vi "database_connection_write_dev_MQTT_no_database.vi"(5 "ODBC data source name":string="amrc_monitoring", 6 "error in (no error)":errorcluster, 7 "G1?":u32, 8 "current time":timestamp, 9 "data 2":dbl[](array[numeric]), 10 "Machine Data":T4={"Zload"="", "Yload"="", "Xload"="", "path_position"="", "Fovr"="", "SspeedOvr"="", "Program Name"="", "Program status"="", "Block of code being executed"="", "Line of code"="", "Machine availability"="", "Emergency status"="", "Controller mode"="", "Tool_id"="UNAVAILABLE"}, 11 "Machine type":string) -> (3 "error out":errorcluster)   [LabVIEW 2017]
uses:
  <vilib>/regexp/Match Regular Expression.xnode
  mqtt Folder/src/class/mqtt/mqtt.lvclass
  mqtt Folder/src/class/mqtt/mqttTXqueue/mqttTXdataQueueFunction.ctl
  mqtt Folder/src/class/mqtt/mqttConfigFunction.ctl
  mqtt Folder/src/class/mqtt/mqttTXqueue/mqttRXsubscriptionEventFunction.ctl
  mqtt Folder/src/class/mqtt/mqttTypedef/mqttBroker.ctl
  mqtt Folder/src/class/mqtt/mqttTypedef/mqttConnectionFlags.ctl
  mqtt Folder/src/class/mqtt/mqttTypedef/mqttWillInformation.ctl
  <vilib>/addons/database/NI_Database_API.lvlib
  mqtt Folder/src/class/mqtt/mqttTypedef/mqttQOSlevel.ctl
  mqtt Folder/src/class/mqtt/mqttTypedef/mqttConnectionMeta.ctl
  mqtt Folder/src/class/mqtt/mqttTypedef/mqttConnectionStatus.ctl
panel:
  out "error out 3":errorcluster
  out "publishSuccess 2":bool=TRUE
  out "publishMessageID 2":u16 format="%02x"
  out "valueSent 2":string="14:19:17.238_"
  in  "connMeta 2":T1
  in  "topic 2":string="a/b"
  out "connStatus 2":T3
  out "sessionPresent 2":bool
  out "string":string="(timestamp,machine_status,g1,tool_id,force_acc_raw_data,spike_raw_data,spindle_load,spindle_speed,feed_rate,I,J,K,X,Y,Z,position_A,position_B ,Xload,Yload,Zload,Aload,Bload,program_number,accel_x_rms,accel_y_rms,accel_z_rms,force_x_rms,force_y_rms,force_z_rms,axial_force_rms, torque_rms,bending_x_rms,bending_y_rms,estop,block_code,fovr,sspeedovr,program_name,line) VALUES ("
  out "data 3":dbl[](array[numeric])
  out "path_position":string
  out "x = y?":bool
  out "submatch 1":string
  out "after match 3":string
  out "empty? 2":bool
  out "after match 2":string
  out "resulting string 4":string
  out "Xload":string
  out "concatenated string 6":string
  out "resulting string 3":string
  out "concatenated string 2":string
  out "resulting string 2":string
  out "ODBC data source name 2":string="amrc_monitoring"
  out "resulting string":string
  out "size(s)":i32
  out "concatenated string 5":string
  out "concatenated string 3":string
  out "concatenated string":string
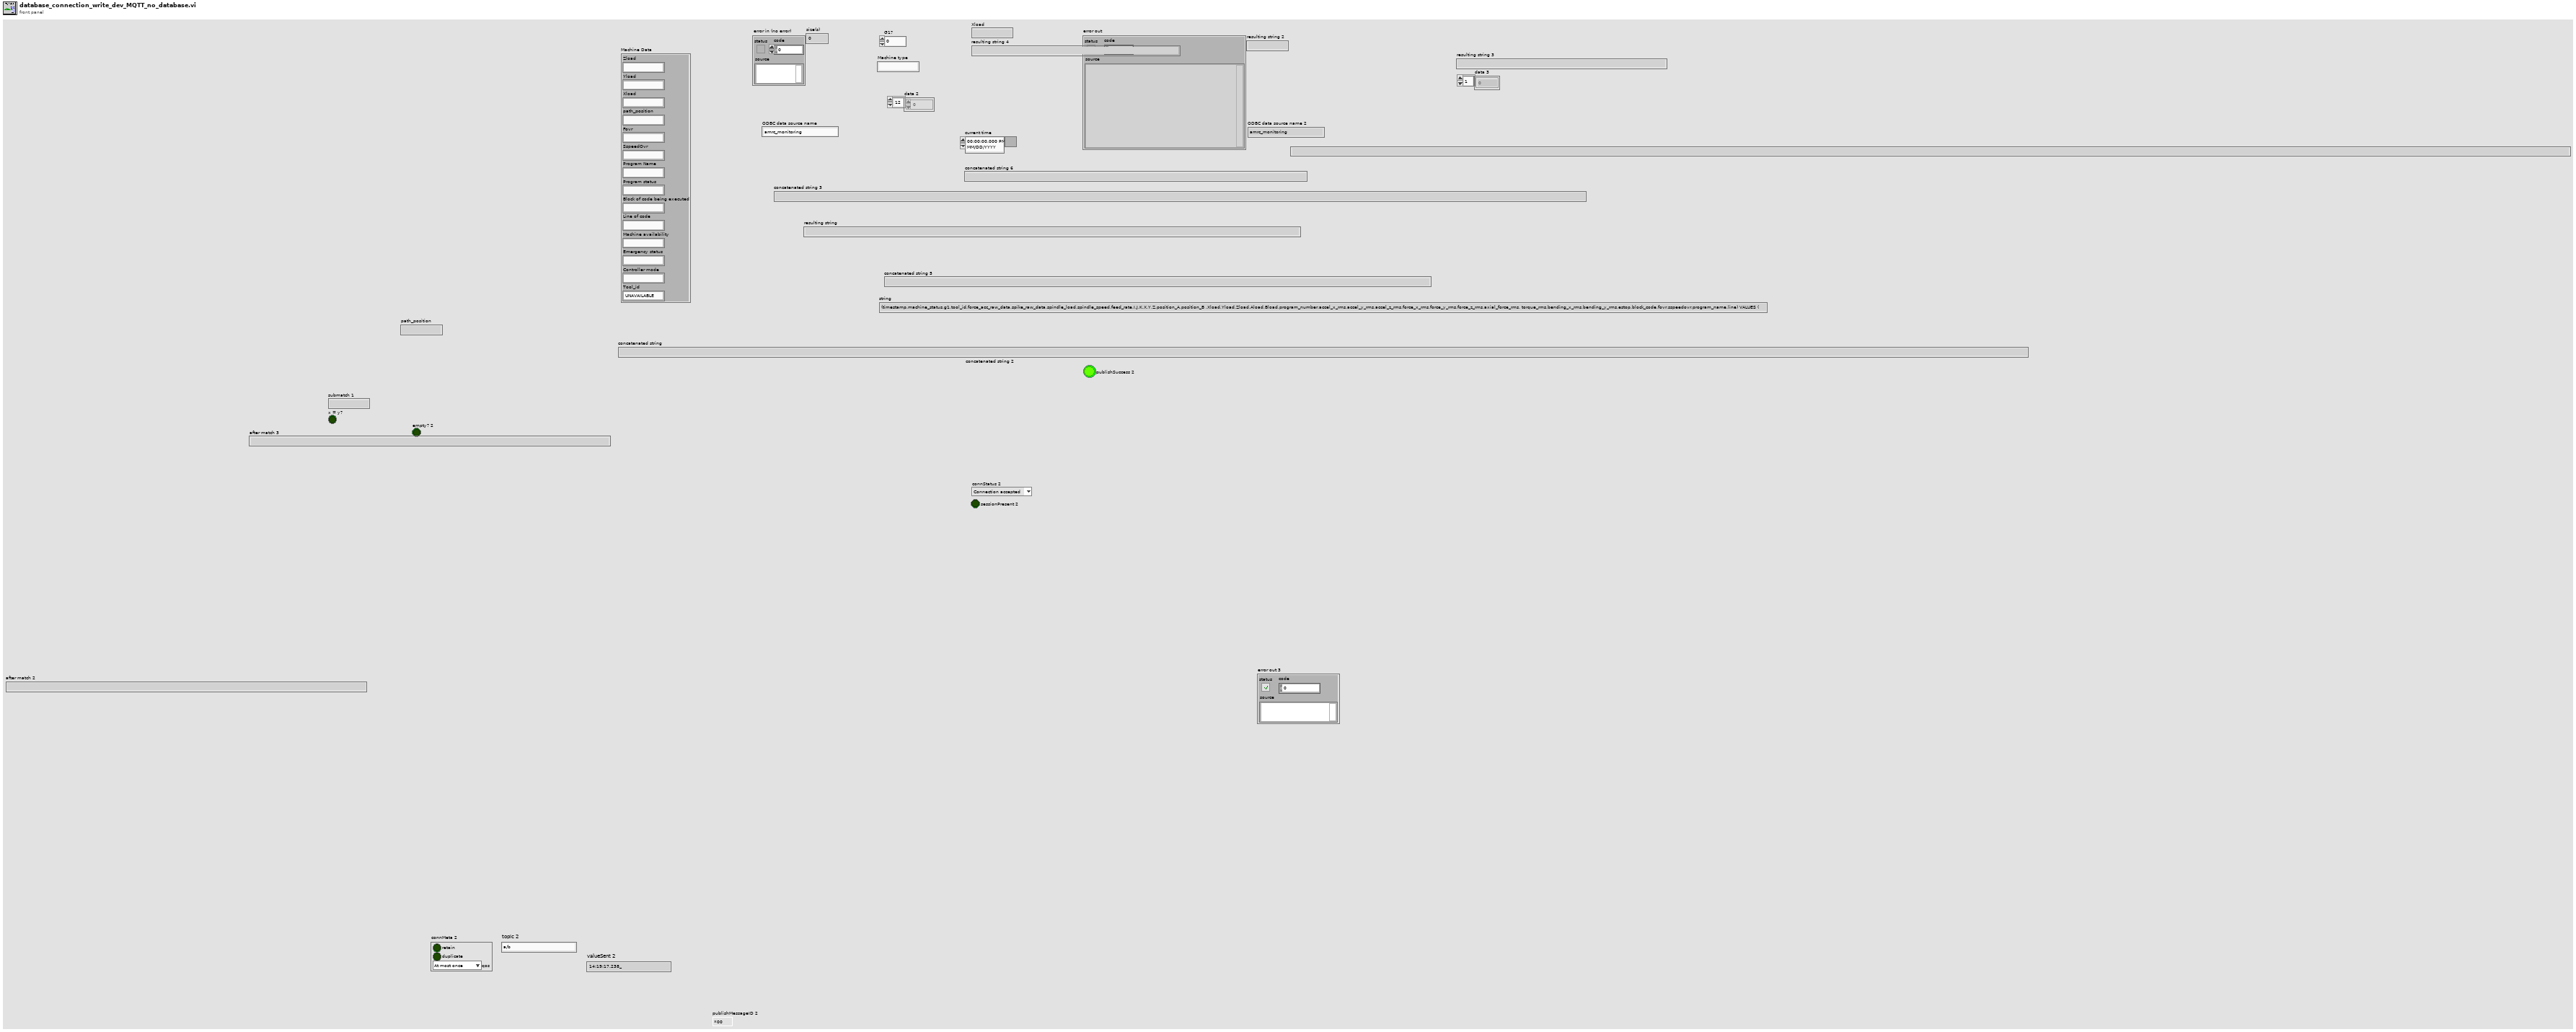
[diagram p1: front panel]
types:
  T1 = typedef "mqttConnectionMeta.ctl" = cluster{"retain":bool, "duplicate":bool, "qos":T2}
  T2 = typedef "mqttQOSlevel.ctl" = enum8{"At most once", "At least once", "Exactly once", "Reserved"}
  T3 = typedef "mqttConnectionStatus.ctl" = enum16{"Connection accepted", "Connection refused: unacceptable protocol version", "Connection refused: identifier rejected", "Connection refused: Server unavailable", "Connection refused: bad user name or password", "Connection refused: not authorized"}
  T4 = cluster{"Zload":string, "Yload":string, "Xload":string, "path_position":string, "Fovr":string, "SspeedOvr":string, "Program Name":string, "Program status":string, "Block of code being executed":string, "Line of code":string, "Machine availability":string, "Emergency status":string, "Controller mode":string, "Tool_id":string}
  T5 = typedef "mqttRXsubscriptionEventFunction.ctl" = enum16{"init", "deinit", "getEventRef", "event"}
  T6 = typedef "mqttTXdataQueueFunction.ctl" = enum16{"init", "deinit", "getQueue", "enqueue"}
  T7 = typedef "mqttWillInformation.ctl" = cluster{"User Name":string, "Password":string}
  T8 = typedef "mqttConnectionFlags.ctl" = cluster{"reserved":bool, "clean session":bool, "will flag":bool, "willQOS":enum8{"At most once", "At least once", "Exactly once", "Reserved"}, "will retain":bool, "password":bool, "user name":bool}
  T9 = typedef "mqttBroker.ctl" = cluster{"address":string, "port":u16, "connTimeout":i32, "writeTimeout":i32, "readTimeout":i32, "subTimeout":i32}
  T10 = typedef "mqtt.lvclass/mqttConfigFunction.ctl" = enum16{"init", "deinit", "set", "get"}
  T11 = enum8{"Enabled", "Disabled", "Disabled and Grayed Out"}
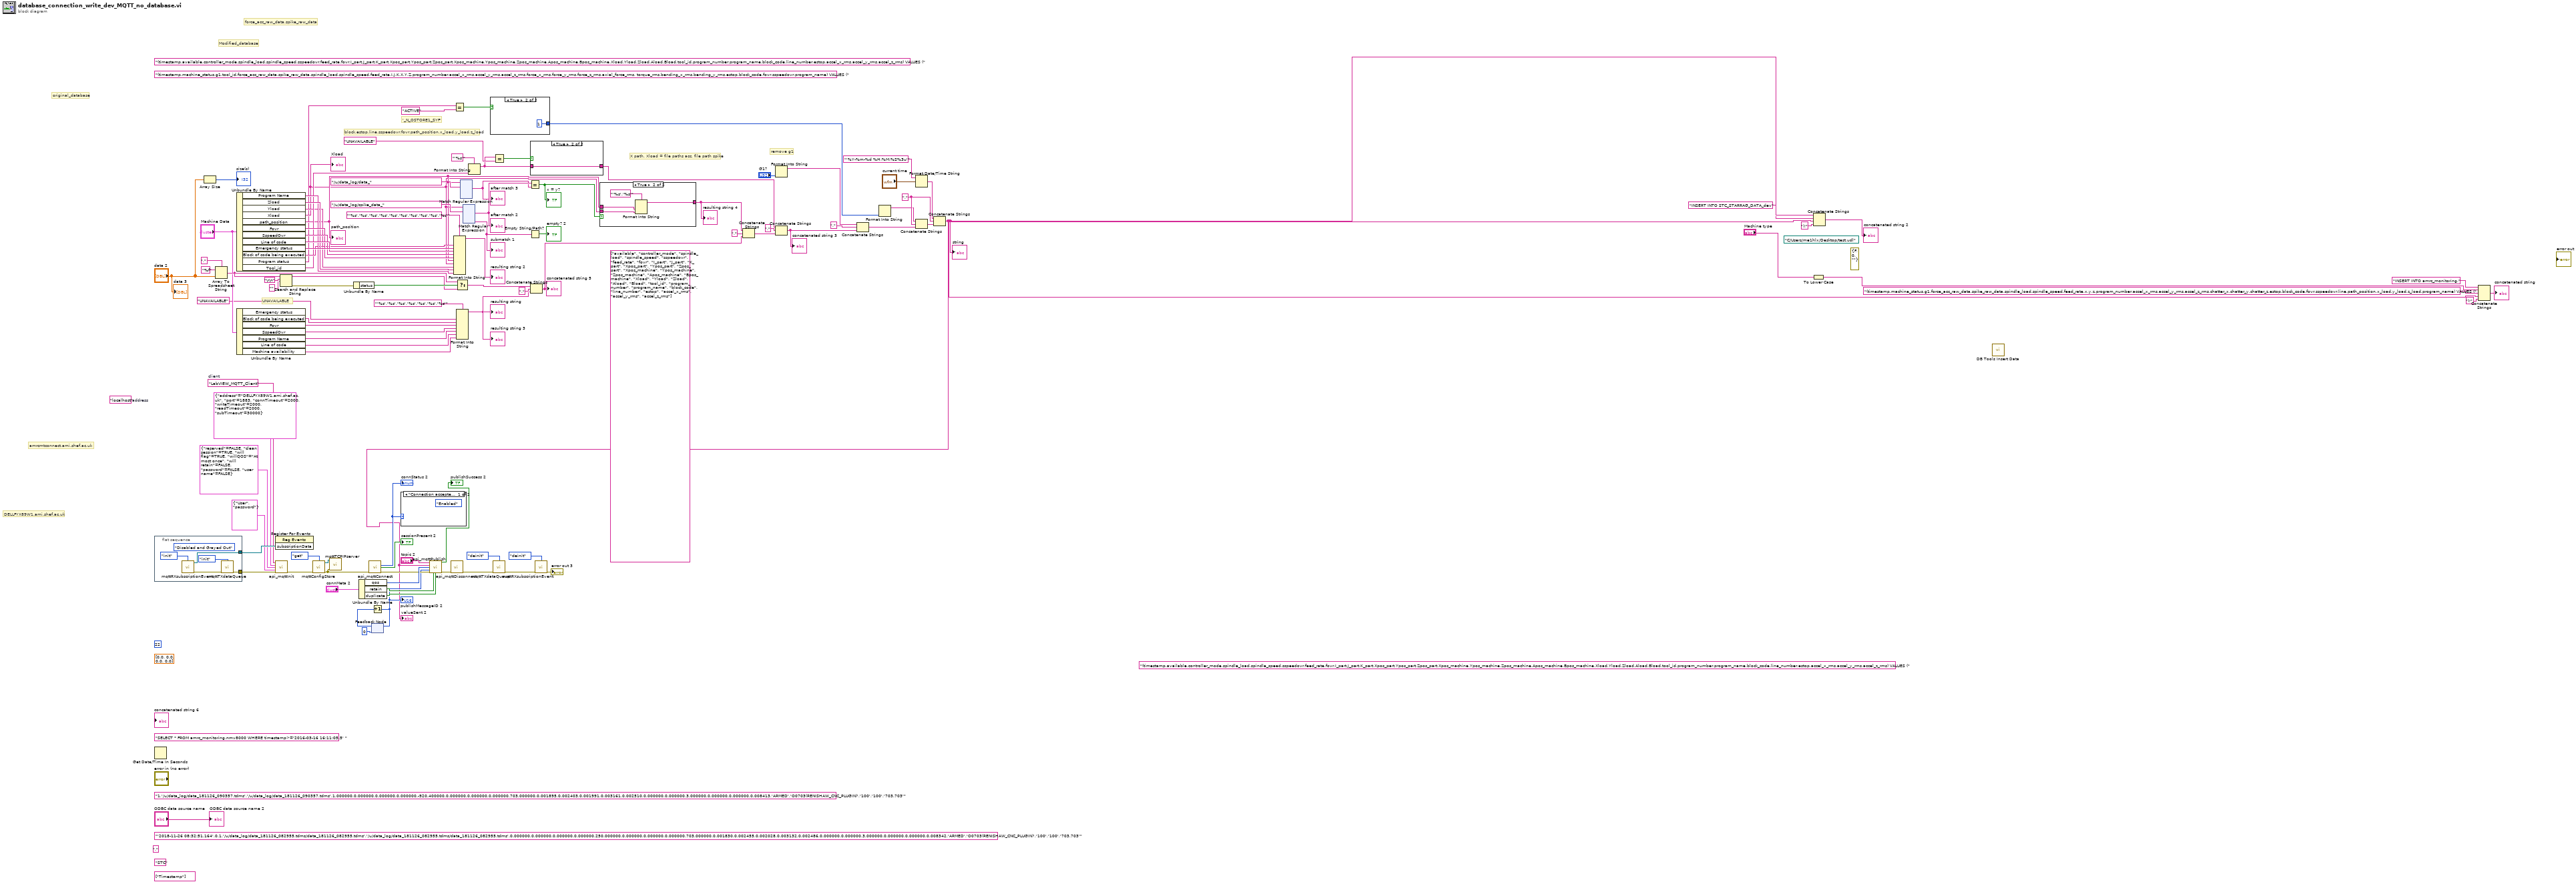
[diagram p0: block diagram]
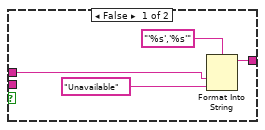
[diagram p3: hidden frame]
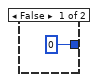
[diagram p5: hidden frame]
diagram:
  (unwired) string[] ["available", "controller_mode", "spindle_load", "spindle_speed", "sspeedovr", "feed_rate", "fovr", "I_part", "J_part", "K_part", "Xpos_part", "Ypos_part", "Zpos_part", "Xpos_machine", "Ypos_machine", "Zpos_machine", "Apos_machine", "Bpos_machine", "Xload", "Yload", "Zload", "Aload", "Bload", "tool_id", "program_number", "program_name", "block_code", "line_number", "estop", "accel_x_rms", "accel_y_rms", "accel_z_rms"]
  (unwired) "(timestamp,available,controller_mode,spindle_load,spindle_speed,sspeedovr,feed_rate,fovr,I_part,J_part,K_part,Xpos_part,Ypos_part,Zpos_part,Xpos_machine,Ypos_machine,Zpos_machine,Apos_machine,Bpos_machine,Xload,Yload,Zload,Aload,Bload,tool_id,program_number,program_name,block_code,line_number,estop,accel_x_rms,accel_y_rms,accel_z_rms) VALUES (" ("string")
  (unwired) "(timestamp,available,controller_mode,spindle_load,spindle_speed,sspeedovr,feed_rate,fovr,I_part,J_part,K_part,Xpos_part,Ypos_part,Zpos_part,Xpos_machine,Ypos_machine,Zpos_machine,Apos_machine,Bpos_machine,Xload,Yload,Zload,Aload,Bload,tool_id,program_number,program_name,block_code,line_number,estop,accel_x_rms,accel_y_rms,accel_z_rms) VALUES (" ("string")
  (unwired) "localhost"  # address
  w25 = "LabVIEW_MQTT_Client"  # client
  (unwired) "(timestamp,machine_status,g1,tool_id,force_acc_raw_data,spike_raw_data,spindle_load,spindle_speed,feed_rate,I,J,K,X,Y,Z,program_number,accel_x_rms,accel_y_rms,accel_z_rms,force_x_rms,force_y_rms,force_z_rms,axial_force_rms, torque_rms,bending_x_rms,bending_y_rms,estop,block_code,fovr,sspeedovr,program_name) VALUES (" ("string")
  (unwired) dbl[] [0.0, 0.0, 0.0, 0.0]
  (unwired) "1,'/u/data_log/data_181126_090357.tdms','/u/data_log/data_181126_090357.tdms',1.000000,0.000000,0.000000,0.000000,-920.400000,0.000000,0.000000,0.000000,703.000000,0.001895,0.002403,0.001991,0.003161,0.002510,0.000000,0.000000,3.000000,0.000000,0.000000,0.008413,'ARMED','O0703(RENISHAW_CNC_PLUGIN)','100','100','703.703'" ("concatenated string 4")
  (unwired) "'2018-11-26 08:32:51.164',0,1,'/u/data_log/data_181126_082955.tdms/data_181126_082955.tdms','/u/data_log/data_181126_082955.tdms/data_181126_082955.tdms',0.000000,0.000000,0.000000,0.000000,250.000000,0.000000,0.000000,0.000000,703.000000,0.001830,0.002455,0.002028,0.003132,0.002486,0.000000,0.000000,3.000000,0.000000,0.000000,0.008342,'ARMED','O0703(RENISHAW_CNC_PLUGIN)','100','100','703.703'" ("concatenated string 2")
  (unwired) 22
  (unwired) errorcluster {"status"=FALSE, "code"=0, "source"=""} ("error in (no error)")
  (unwired) "," ("string")
  (unwired) string[] ["Timestamp"]
  (unwired) "STC"
  (unwired) path "C:/Users/me1hlx/Desktop/test.udl" ("connection information")
  w67 = "," ("string")
  (unwired) "SELECT * FROM amrc_monitoring.nmv8000 WHERE timestamp>='2016-03-16 16:11:05.5' " ("SQL query")
  # "original_database"
  # "X path, Xload = file paths acc, file path spike"
  # "remove g1"
  # "force_acc_raw_data,spike_raw_data"
  # "Modified_database"
  # "amrcmtconnect.ami.shef.ac.uk"
  # "DELLFYX89W1.ami.shef.ac.uk"
  # "'_N_OSTORE1_SYF'"
  # "UNAVAILABLE"
  # "block,estop,line,sspeedovr,fovr,path_position,x_load,y_load,z_load"
  n1 = flat-sequence {
    tunnel: [w110] -> w30
    tunnel: [w107] -> w26
    frame #0 {
      (unwired) T11."Disabled and Grayed Out" ("Disabled")
      n2 = call "mqttRXsubscriptionEvent.vi"("function"=mqttRXsubscriptionEventFunction."init") -> ("subscriptionData"=w107:refnum<user-event>, "error out"=w109:errorcluster)  [unwired: 13 in]
      n3 = call "mqttTXdataQueue.vi"("function"=mqttTXdataQueueFunction."init", "error in (no error)"=w109) -> ("error out"=w110:errorcluster)  [unwired: 12 in, 1 out]
    }
  }
  n4 = Get Date/Time In Seconds() -> ()  [unwired: 1 out]
  n5 = Array Size(array="data 2") -> (size(s)=→"size(s)":i32)
  n6 = Array To Spreadsheet String(delimiter (Tab)=",", array="data 2", 3:"%f" ("format string")) -> (spreadsheet string=w92:string)
  n7 = Unbundle By Name("Machine Data") -> ("Program Name"=w79:string, "Zload"=w83:string, "Yload"=w53:string, "Xload"=w35:string, "path_position"=w36:string, "Fovr"=w84:string, "SspeedOvr"=w85:string, "Line of code"=w86:string, "Emergency status"=w87:string, "Block of code being executed"=w77:string, "Program status"=w2:string, "Tool_id"=w71:string)
  "Xload" <- w35
  "path_position" <- w36
  n8 = Unbundle By Name("Machine Data") -> ("Block of code being executed"=w60:string, "Fovr"=w59:string, "SspeedOvr"=w58:string, "Program Name"=w57:string, "Line of code"=w33:string, "Machine availability"=w31:string)  [unwired: 1 out]
  n9 = register-events(w26) -> ()  [unwired: 2 in, 2 out]
  n10 = call "api_mqttInit.vi"("client"=w25, "broker"=T9 {"address"="DELLFYX89W1.ami.shef.ac.uk", "port"=1883, "connTimeout"=2000, "writeTimeout"=2000, "readTimeout"=2000, "subTimeout"=30000}, "connFlags"=T8 {"reserved"=FALSE, "clean session"=TRUE, "will flag"=TRUE, "willQOS"=enum."At most once", "will retain"=FALSE, "password"=FALSE, "user name"=FALSE}, "User Info"=T7 {"User Name"="User", "Password"="password"}, "error in (no error)"=w30) -> ("error out"=w28:errorcluster)  [unwired: 10 in]
  n11 = Search and Replace String(input string=w92, search string="\r\n", replace string="" ("replace string (\"\")")) -> (result string=w93:string, error out=w95:errorcluster)  [unwired: 5 in, 2 out]
  n12 = call "mqttConfigStore.vi"("function"=mqttConfigFunction."get", "error in (no error)"=w28) -> ("mqtt.lvclass out"=w27:refnum<class "mqtt.lvclass">, "error out"=w19:errorcluster)  [unwired: 12 in]
  n13 = call "mqttTCPIPserver.vi"("mqtt.lvclass"=w27, "error in (no error)"=w19) -> ()  [unwired: 12 in, 2 out]
  n14 = Unbundle By Name(w95) -> ("status"=w94:bool)
  n15 = Unbundle By Name("connMeta 2") -> ("qos"=w16:T2, "retain"=w15:bool, "duplicate"=w14:bool)
  n16 = call "api_mqttConnect.vi"("error in (no error)"=w19) -> ("connStatus"=w21:T3, "sessionPresent"=→"sessionPresent 2":bool, "error out"=w13:errorcluster)  [unwired: 11 in, 1 out]
  "connStatus 2" <- w21
  n17 = feedback #1(u16 0) -> (w11:u16)
  n18 = Increment(x=w11) -> (x+1=w10:u16)
  "publishMessageID 2" <- w10
  n19 = feedback-in #1(w10) -> ()
  n20 = case shown="\"Connection accepted\"" w21 {
    frame "Connection accepted" {
      (unwired) T11."Enabled" ("Disabled")
    }
    frame Default {
    }
  }
  n21 = Format Into String(format string="'%s','%s','%s','%s','%s','%s','%s','%s','%s','%s'", w77, w87, w86, w85, w84, w36, w35, w53, w83, w79) -> (resulting string=→"resulting string 2":string)  [unwired: 2 in, 1 out]
  n22 = Equal?(x=w2, y="ACTIVE") -> (x = y?=w103:bool)
  n23 = Select(t=w92, s=w94, f=w93) -> (s? t:f=w80:string)
  n24 = Format Into String(format string="'%s','%s','%s','%s','%s','%s','%s'", "UNAVAILABLE" ("format string"), w60, w59, w58, w57, w33, w31) -> (resulting string=w52:string)  [unwired: 2 in, 1 out]
  "resulting string" <- w52
  "resulting string 3" <- w52
  n25 = xnode "Match Regular Expression"("input string"=w36, "regular expression"="/u/data_log/data_") -> ("after match"=w38:string)  [unwired: 4 in, 5 out]
  "after match 3" <- w38
  n26 = xnode "Match Regular Expression"("input string"=w35, "regular expression"="/u/data_log/spike_data_") -> ("after match"=w39:string, "submatch 1"=w40:string)  [unwired: 4 in, 4 out]
  "after match 2" <- w39
  "submatch 1" <- w40
  n27 = Format Into String(format string="'%s'", w71) -> (resulting string=w70:string)  [unwired: 2 in, 1 out]
  n28 = case shown="True" w103 {
    tunnel: [0 1] -> w49
    frame False {
    }
    frame True {
    }
  }
  n29 = Equal?(x=w70, y="UNAVAILABLE") -> (x = y?=w102:bool)
  n30 = Equal?(x=w39, y=w38) -> (x = y?=w37:bool)
  "x = y?" <- w37
  n31 = Empty String/Path?(string/path=w40) -> (empty?=→"empty? 2":bool)
  n32 = case shown="True" w102 {
    tunnel: w70 -> [w114 w115]
    tunnel: [w114 w115] -> w32
    frame False {
    }
    frame True {
    }
  }
  n33 = Concatenate Strings(w80, "," ("string"), w52) -> (w47:string)
  "concatenated string 5" <- w47
  n34 = case shown="True" w37 {
    tunnel: w36 -> [w118 w120]
    tunnel: w35 -> [_ w123]
    tunnel: [w117 w121] -> w34
    frame False {
      n35 = Format Into String(format string="'%s','%s'", w118, "Unavailable" ("Tool_id")) -> (resulting string=w117:string)  [unwired: 2 in, 1 out]
    }
    frame True {
      n36 = Format Into String(format string="'%s','%s'", w120, w123) -> (resulting string=w121:string)  [unwired: 2 in, 1 out]
    }
  }
  "resulting string 4" <- w34
  n37 = Concatenate Strings(w34, "," ("string"), w47) -> (w45:string)
  n38 = Format Into String("G1?") -> (resulting string=w65:string)  [unwired: 3 in, 1 out]
  n39 = Concatenate Strings(w32, "," ("string"), w45) -> (w50:string)
  "concatenated string 3" <- w50
  n40 = Concatenate Strings(w65, "," ("string"), w50) -> (w51:string)
  n41 = Format Into String(w49) -> (resulting string=w66:string)  [unwired: 3 in, 1 out]
  n42 = Format Date/Time String(time format string (%c)="'%Y-%m-%d %H:%M:%S%3u'", seconds (now)="current time") -> (date/time string=w68:string)  [unwired: 1 in]
  n43 = Concatenate Strings(w66, w67, w51) -> (w98:string)
  n44 = Concatenate Strings(w68, w67, w98) -> (w1:string)
  "string" <- w1
  "valueSent 2" <- w1
  n45 = call "api_mqttPublish.vi"("topic"="topic 2", "value"=w1, "QoS (At most once)"=w16, "messageID"=w10, "error in (no error)"=w13, "retain(F)"=w15, "duplicate(F)"=w14) -> ("success"=→"publishSuccess 2":bool, "error out"=w3:errorcluster)  [unwired: 7 in]
  n46 = call "api_mqttDisconnect.vi"("error in (no error)"=w3) -> ("error out"=w7:errorcluster)  [unwired: 13 in, 1 out]
  n47 = call "mqttTXdataQueue.vi"("function"=mqttTXdataQueueFunction."deinit", "error in (no error)"=w7) -> ("error out"=w5:errorcluster)  [unwired: 12 in, 1 out]
  n48 = call "mqttRXsubscriptionEvent.vi"("function"=mqttRXsubscriptionEventFunction."deinit", "error in (no error)"=w5) -> ("error out"=→"error out 3":errorcluster)  [unwired: 12 in, 1 out]
  n49 = To Lower Case(string="Machine type") -> (all lower case string=w89:string)
  n50 = Concatenate Strings("INSERT INTO STC_STARRAG_DATA_dev" ("string"), w1, w1, ");" ("string")) -> (→"concatenated string 2":string)
  n51 = call <vilib>:"DB Tools Insert Data.vi"() -> ()  [unwired: 10 in, 2 out]
  n52 = Concatenate Strings("INSERT INTO amrc_monitoring." ("string"), w89, "(timestamp,machine_status,g1,force_acc_raw_data,spike_raw_data,spindle_load,spindle_speed,feed_rate,x,y,z,program_number,accel_x_rms,accel_y_rms,accel_z_rms,chatter_x,chatter_y,chatter_z,estop,block_code,fovr,sspeedovr,line,path_position,x_load,y_load,z_load,program_name) VALUES (" ("string"), w1, ");" ("string")) -> (→"concatenated string":string)
  "ODBC data source name 2" <- "ODBC data source name"
  "data 3" <- "data 2"
